vi "replaceNameToken.vi"(8 "error in (no error)":errorcluster, 10 "Query In":string, 11 "Category in":refnum<class "Category.lvclass">) -> (0 "error out":errorcluster, 2 "Query Out":string, 3 "Category out":refnum<class "Category.lvclass">)   [LabVIEW 2020, in "Category.lvclass"]
uses:
  Category.lvclass
  Category.lvclass/Category.ctl
  UserEditableAmount/UserEditableAmount.lvclass
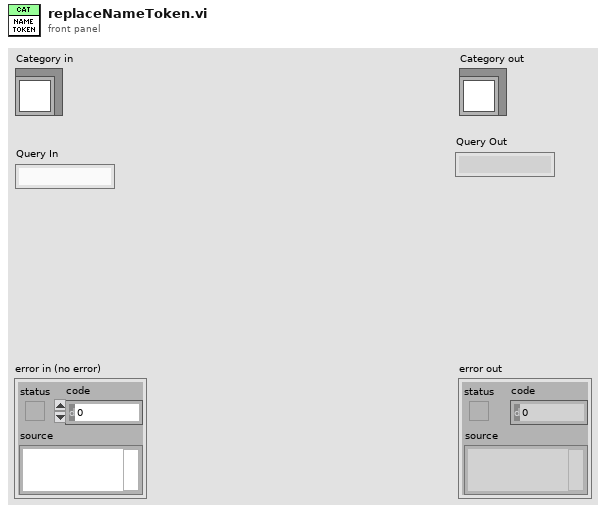
[diagram p1: front panel]
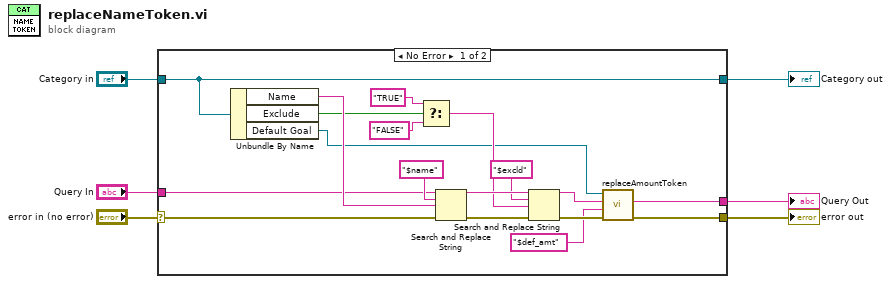
[diagram p0: block diagram]
diagram:
  n1 = case shown="No Error" "error in (no error)" {
    selector: "error in (no error)" -> [w22 w26]
    tunnel: [w11 w26] -> w5
    tunnel: [w23 w25] -> w3
    tunnel: "Category in" -> [w23 w25]
    tunnel: "Query In" -> [w20 _]
    tunnel: [w10 _] -> w1
    frame No Error {
      n2 = Unbundle By Name(w23) -> ("Name"=w21:string, "Exclude"=w15:bool, "Default Goal"=w8:refnum<class "UserEditableAmount.lvclass">)
      n3 = Select(t="TRUE", s=w15, f="FALSE") -> (s? t:f=w13:string)
      n4 = Search and Replace String(input string=w20, search string="$name", replace string=w21, error in=w22) -> (result string=w19:string, error out=w18:errorcluster)  [unwired: 4 in, 2 out]
      n5 = Search and Replace String(input string=w19, search string="$excld", replace string=w13, error in=w18) -> (result string=w9:string, error out=w12:errorcluster)  [unwired: 4 in, 2 out]
      n6 = call "replaceAmountToken.vi"("error in (no error)"=w12, "amt token"="$def_amt", "Query In"=w9, "UserEditableAmount in"=w8) -> ("error out"=w11:errorcluster, "Query Out"=w10:string)  [unwired: 5 in, 1 out]
    }
    frame Error {
    }
  }
  "error out" <- w5
  "Category out" <- w3
  "Query Out" <- w1
